vi "Get Section.vi"(11 "File Info in":refnum<class "File Info.lvclass">) -> (2 "Section":string, 3 "File Info out":refnum<class "File Info.lvclass">)   [LabVIEW 2024, in "EDS.lvlib" / "File Info.lvclass"]
uses:
  File Info.lvclass
  File Info.lvclass/File Info.ctl
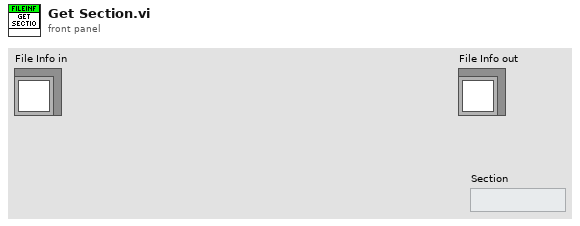
[diagram p1: front panel]
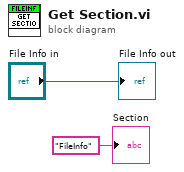
[diagram p0: block diagram]
diagram:
  "File Info out" <- "File Info in"
  "Section" <- "FileInfo" ("Section")
